vi "projector validation.vi"(0 "Image Src":T1, 1 "blue channel":T1, 4 "on/off level":dbl, 5 "error in (no error)":errorcluster) -> (16 "on/off":bool, 19 "error out":errorcluster)   [LabVIEW 2019]
uses:
  <vilib>/vision/Image Controls.llb/IMAQ Image.ctl
  <vilib>/vision/NI_Vision_Development_Module.lvlib
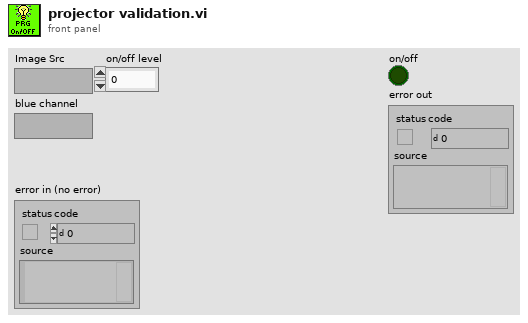
[diagram p1: front panel]
types:
  T1 = typedef "IMAQ Image.ctl" = refnum<image>
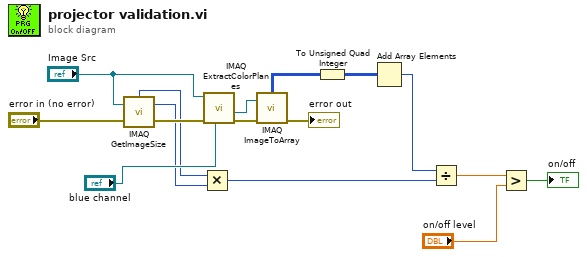
[diagram p0: block diagram]
diagram:
  n1 = call "IMAQ GetImageSize"("Image"="Image Src", "error in (no error)"="error in (no error)") -> ("Y Resolution"=w4:i32, "X Resolution"=w3:i32, "error out"=w5:errorcluster)  [unwired: 2 in]
  n2 = Multiply(x=w3, y=w4) -> (x*y=w11:i32)
  n3 = call "IMAQ ExtractColorPlanes"("Blue or Luma or Val or Inten Plane"="blue channel", "error in (no error)"=w5, "Image Src"="Image Src") -> ("error out"=w7:errorcluster, "Blue or Luma or Val or Inten Plane out"=w16:T1)  [unwired: 5 in, 2 out]
  n4 = call "IMAQ ImageToArray"("error in (no error)"=w7, "Image"=w16) -> ("error out"=→"error out":errorcluster, "Image Pixels (U8)"=w15:u8[][])  [unwired: 2 in, 3 out]
  n5 = To Unsigned Quad Integer(1:w15) -> (0:w14:u64[][])
  n6 = Add Array Elements(numeric array=w14) -> (sum=w13:u64)
  n7 = Divide(x=w13, y=w11) -> (x/y=w10:dbl)
  n8 = Greater?(x=w10, y="on/off level") -> (0:→"on/off":bool)
